vi "ParsePacket.vi"(11 "Buffer":u8[](array[numeric])) -> (2 "Ok?":bool, 3 "Packet":T1)   [LabVIEW 2009]
uses:
  Packet.ctl
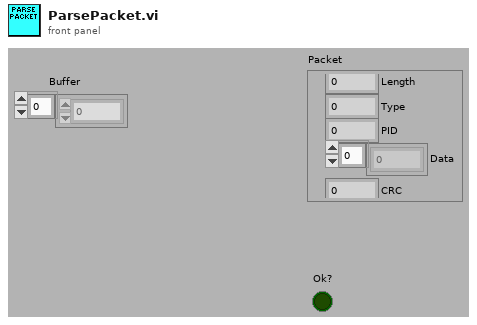
[diagram p1: front panel]
types:
  T1 = typedef "Packet.ctl" = cluster{"Length":u8, "Type":u8, "PID":u8, "Data":u8[], "CRC":u8}
  T2 = cluster{"Length":u8, "Type":u8, "PID":u8, "Data":u8[], "CRC":u8}
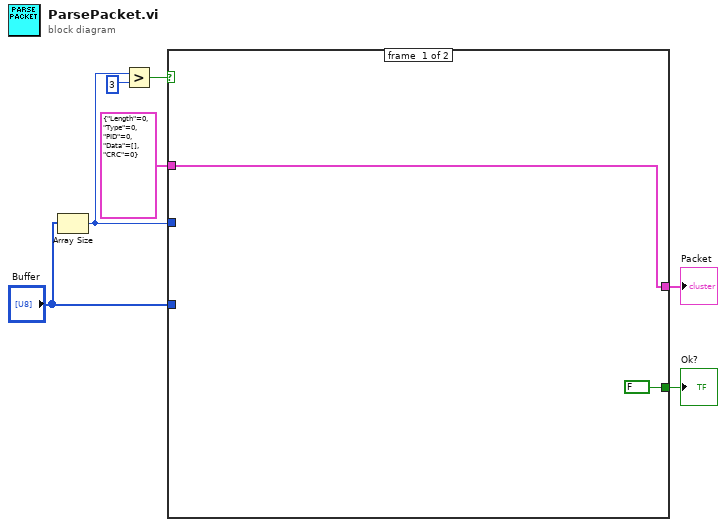
[diagram p0: block diagram]
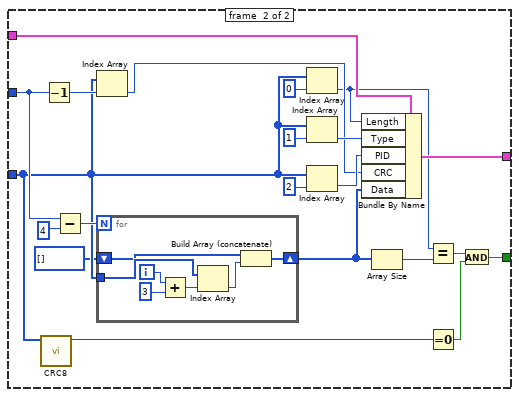
[diagram p2: hidden frame]
diagram:
  n1 = Array Size(array="Buffer") -> (size(s)=w3:i32)
  n2 = Greater?(x=w3, y=3) -> (0:w4:bool)
  n3 = case shown="True" w4 {
    tunnel: [w9 w23] -> w1
    tunnel: T2 {"Length"=0, "Type"=0, "PID"=0, "Data"=[], "CRC"=0} ("Packet") -> [w9 w22]
    tunnel: "Buffer" -> [_ w17]
    tunnel: w3 -> [_ w20]
    tunnel: [FALSE w10] -> w2
    frame #0 {
    }
    frame #1 {
      n4 = call "CRC8.vi"("Data"=w17) -> ("CRC8"=w21:u8)  [unwired: 10 in]
      n5 = Decrement(x=w20) -> (x-1=w27:i32)
      n6 = Subtract(x=w20, y=4) -> (x-y=w18:i32)
      n7 = Index Array(array=w17, index=w27) -> (element=w28:u8)
      n8 = for {
        N: w18 -> [_]
        tunnel: w17 -> [w37]
        shift-right: [w32] -> w13
        shift-left: u8[] [] ("Data") -> [w33]
        i -> [w35]
        n9 = Add(x=w35, y=3) -> (x+y=w36:i32)
        n10 = Index Array(array=w37, index=w36) -> (element=w31:u8)
        n11 = Build Array (concatenate)(w33, w31) -> (w32:u8[])
      }
      n12 = Index Array(array=w17, index=0) -> (element=w15:u8)
      n13 = Index Array(array=w17, index=1) -> (element=w30:u8)
      n14 = Index Array(array=w17, index=2) -> (element=w29:u8)
      n15 = Bundle By Name(cluster=w22, "Length"=w15, "Type"=w30, "PID"=w29, "CRC"=w28, "Data"=w13) -> (w23:T2)
      n16 = Array Size(array=w13) -> (size(s)=w14:i32)
      n17 = Equal?(x=w15, y=w14) -> (x = y?=w12:bool)
      n18 = Equal To 0?(x=w21) -> (x = 0?=w11:bool)
      n19 = And(x=w12, y=w11) -> (x .and. y?=w10:bool)
    }
  }
  "Ok?" <- w2
  "Packet" <- w1
